vi "fp4task2.vi"   [LabVIEW 2016]
uses:
  <vilib>/NXT/Block Support/NXT_InputPort.ctl
  <vilib>/NXT/Block Support/NXT_OutputPort.ctl
  <vilib>/NXT/NXTIO Xnodes/NXTIONodeSubVIs/LEGOResetMotors.vi
  <vilib>/NXT/Dual Mode Library/Waits/Wait_Bump.vi
  <vilib>/NXT/Dual Mode Library/Sensors/EV3_Ultrasonic_CM.vi
  <vilib>/NXT/Dual Mode Library/Sensors/Touch_Pressed.vi
  <vilib>/NXT/NXTIO Xnodes/NXTIONodeSubVIs/NXTMoveMotors.vi
  <vilib>/NXT/NXTIO Xnodes/NXTIONodeSubVIs/NXTMotorRunDistance.vi
  <vilib>/NXT/NXTIO Xnodes/NXTIONodeSubVIs/LEGOStopAllMotors.vi
  <vilib>/NXT/Dual Mode Library/Sound/Tone.vi
  <vilib>/NXT/Dual Mode Library/Waits/Wait_Num.vi
  <vilib>/NXT/Dual Mode Library/Sound/PlayA.vi
  <vilib>/NXT/Subs/LVHSConnector.ctl
  <vilib>/NXT/NXTIO Xnodes/AddressXNode/NXTIOAddress.xnode
  <vilib>/NXT/NXTIO Xnodes/NXTIOXNode/NXTIO.xnode
  <vilib>/NXT/LegoClasses/BrickReference/BrickReference.lvclass
types:
  T1 = typedef "NXT_OutputPort.ctl" = u8
  T2 = typedef "NXT_InputPort.ctl" = u32
  T3 = typedef "LVHSConnector.ctl" = refnum<class "BrickReference.lvclass">
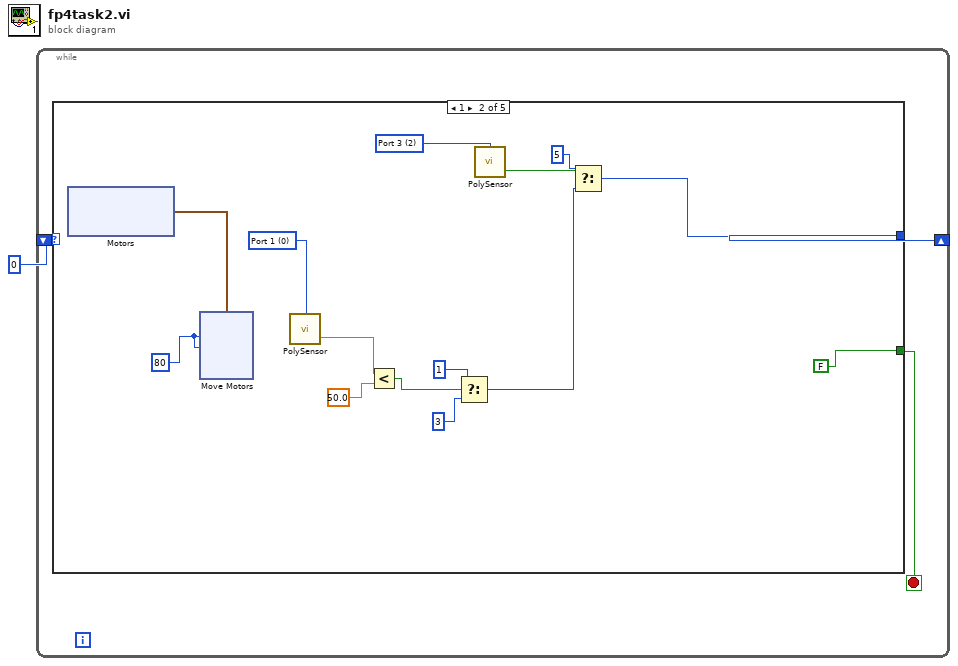
[diagram p0: block diagram]
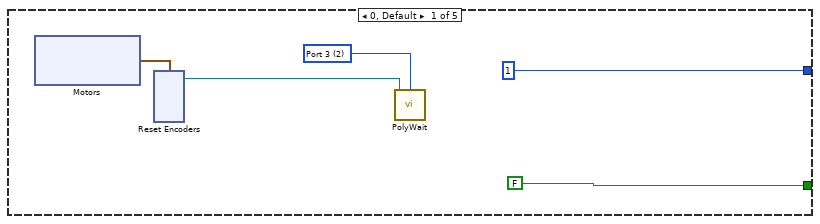
[diagram p2: hidden frame]
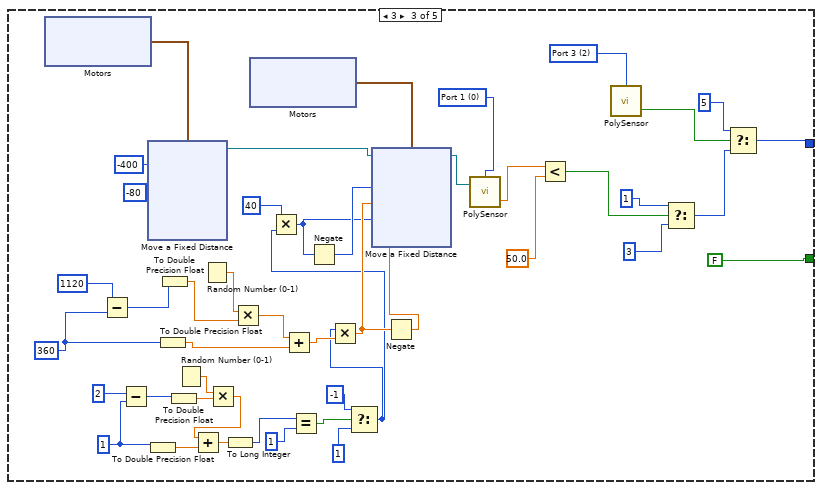
[diagram p3: hidden frame]
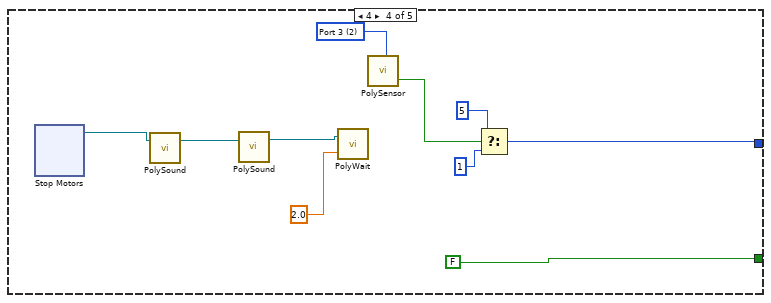
[diagram p4: hidden frame]
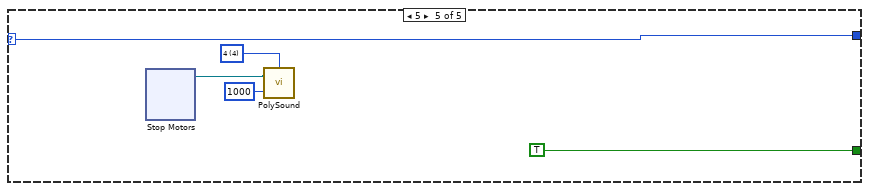
[diagram p5: hidden frame]
diagram:
  n1 = while {
    shift-right: [w4] -> _
    shift-left: 0 -> [w3]
    stop <- w2 stop-if-true
    n2 = case shown="1" w3 {
      selector: w3 -> [_ _ _ _ w126]
      tunnel: [1 w27 w82 w111 w126] -> w4
      tunnel: [FALSE FALSE FALSE FALSE TRUE] -> w2
      frame 0, Default {
        w6 = T2 2 items=["Port 1", "Port 2", "Port 3", "Port 4"] ("Port (Port 1)")
        n3 = xnode "Motors"() -> ("Motor"=w9:cluster{"Port":T1, "Port":T1})
        n4 = xnode "Reset Encoders"("Motors"=w9) -> ("NXT/EV3"=w5:T3)  [unwired: 1 in]
        n5 = call-poly <vilib>:"PolyWait.vi"("NXT/EV3"=w5, "Port (Port 1)"=w6) -> ()  [unwired: 2 in, 1 out]
      }
      frame 1 {
        w18 = 80 ("Distance 1")
        w25 = T2 2 items=["Port 1", "Port 2", "Port 3", "Port 4"] ("Port (Port 1)")
        w16 = T2 0 items=["Port 1", "Port 2", "Port 3", "Port 4"] ("Port (Port 1)")
        n6 = xnode "Motors"() -> ("Motor"=w19:cluster{"Port":T1, "Port":T1})
        n7 = xnode "Move Motors"("Power/Speed 2"=w18, "Power/Speed 1"=w18, "Motors"=w19) -> ()  [unwired: 1 in, 1 out]
        n8 = call-poly <vilib>:"PolySensor.vi"("Port (Port 1)"=w16) -> ("Centimeters"=w15:sgl)  [unwired: 2 in, 1 out]
        n9 = Less?(x=w15, y=sgl 50.0) -> (x < y?=w22:bool)
        n10 = Select(t=1, s=w22, f=3) -> (s? t:f=w17:i32)
        n11 = call-poly <vilib>:"PolySensor.vi"("Port (Port 1)"=w25) -> ("Yes / No"=w24:bool)  [unwired: 2 in, 1 out]
        n12 = Select(t=5, s=w24, f=w17) -> (s? t:f=w27:i32)
      }
      frame 3 {
        w55 = 1
        w66 = 360
        w70 = -80 ("Distance 1")
        w71 = -400 ("Distance 1")
        w60 = T2 0 items=["Port 1", "Port 2", "Port 3", "Port 4"] ("Port (Port 1)")
        w75 = T2 2 items=["Port 1", "Port 2", "Port 3", "Port 4"] ("Port (Port 1)")
        n13 = xnode "Motors"() -> ("Motor"=w72:cluster{"Port":T1, "Port":T1})
        n14 = Subtract(x=1120, y=w66) -> (x-y=w67:i32)
        n15 = Subtract(x=2, y=w55) -> (x-y=w56:i32)
        n16 = xnode "Move a Fixed Distance"("Speed 2"=w70, "Speed 1"=w70, "Distance 2"=w71, "Distance 1"=w71, "Motors"=w72) -> ("NXT/EV3"=w69:T3)  [unwired: 1 in]
        n17 = To Double Precision Float(number=w55) -> (double precision float=w54:dbl)
        n18 = To Double Precision Float(number=w66) -> (double precision float=w62:dbl)
        n19 = To Double Precision Float(number=w67) -> (double precision float=w65:dbl)
        n20 = To Double Precision Float(number=w56) -> (double precision float=w53:dbl)
        n21 = Random Number (0-1)() -> (number: 0 to 1=w52:dbl)
        n22 = Random Number (0-1)() -> (number: 0 to 1=w64:dbl)
        n23 = Multiply(x=w52, y=w53) -> (x*y=w50:dbl)
        n24 = Add(x=w50, y=w54) -> (x+y=w51:dbl)
        n25 = To Long Integer(number=w51) -> (32bit integer=w48:i32)
        n26 = Multiply(x=w64, y=w65) -> (x*y=w63:dbl)
        n27 = xnode "Motors"() -> ("Motor"=w73:cluster{"Port":T1, "Port":T1})
        n28 = Add(x=w63, y=w62) -> (x+y=w44:dbl)
        n29 = Equal?(x=w48, y=1) -> (x = y?=w47:bool)
        n30 = Select(t=-1, s=w47, f=1) -> (s? t:f=w41:i32)
        n31 = Multiply(x=40 ("Distance 1"), y=w41) -> (x*y=w38:i32)
        n32 = Negate(x=w38) -> (-x=w39:i32)
        n33 = Multiply(x=w41, y=w44) -> (x*y=w42:dbl)
        n34 = Negate(x=w42) -> (-x=w43:dbl)
        n35 = xnode "Move a Fixed Distance"("Speed 2"=w38, "Speed 1"=w39, "Distance 2"=w42, "Distance 1"=w43, "Motors"=w73, "NXT/EV3"=w69) -> ("NXT/EV3"=w58:T3)
        n36 = call-poly <vilib>:"PolySensor.vi"("NXT/EV3"=w58, "Port (Port 1)"=w60) -> ("Centimeters"=w59:sgl)  [unwired: 1 in, 1 out]
        n37 = Less?(x=w59, y=50.0) -> (x < y?=w77:bool)
        n38 = call-poly <vilib>:"PolySensor.vi"("Port (Port 1)"=w75) -> ("Yes / No"=w74:bool)  [unwired: 2 in, 1 out]
        n39 = Select(t=1, s=w77, f=3) -> (s? t:f=w80:i32)
        n40 = Select(t=5, s=w74, f=w80) -> (s? t:f=w82:i32)
      }
      frame 4 {
        w110 = T2 2 items=["Port 1", "Port 2", "Port 3", "Port 4"] ("Port (Port 1)")
        n41 = xnode "Stop Motors"() -> ("NXT/EV3"=w118:T3)  [unwired: 2 in]
        n42 = call-poly <vilib>:"PolySound.vi"("NXT/EV3"=w118) -> ("NXT/EV3"=w117:T3)  [unwired: 3 in]
        n43 = call-poly <vilib>:"PolySound.vi"("NXT/EV3"=w117) -> ("NXT/EV3"=w115:T3)  [unwired: 3 in]
        n44 = call-poly <vilib>:"PolyWait.vi"("Time (1 sec)"=sgl 2.0, "NXT/EV3"=w115) -> ()  [unwired: 2 in, 1 out]
        n45 = call-poly <vilib>:"PolySensor.vi"("Port (Port 1)"=w110) -> ("Yes / No"=w109:bool)  [unwired: 2 in, 1 out]
        n46 = Select(t=5, s=w109, f=1) -> (s? t:f=w111:i32)
      }
      frame 5 {
        w123 = u16 4 items=["3"=3, "4"=4, "5"=5, "6"=6, "7"=7] ("Octave")
        n47 = xnode "Stop Motors"() -> ("NXT/EV3"=w124:T3)  [unwired: 2 in]
        n48 = call-poly <vilib>:"PolySound.vi"("Duration (500 ms)"=u16 1000, "NXT/EV3"=w124, "Octave"=w123) -> ()  [unwired: 1 in, 1 out]
      }
    }
  }
